vi "Handle Last Ack Core.vi"(4 "error in (no error)":errorcluster, 6 "Last Ack":refnum<class "Last Ack.lvclass">, 7 "ViewableActor in":refnum<class "ViewableActor.lvclass">) -> (0 "error out":errorcluster, 3 "ViewableActor out":refnum<class "ViewableActor.lvclass">)   [LabVIEW 2020, in "ViewableActor.lvlib" / "ViewableActor.lvclass"]
doc: "(<B>Filename</B>: Actor Framework.lvlib:Actor.lvclass:Handle Last Ack Core.vi)\n\nDefines how the caller actor responds to the Last Ack message from a nested actor. The Last Ack message is the final message a nested actor sends to its caller before it shuts down. The message contains information about the final state of the nested actor.\n\nBy default, this method does nothing except return any error the nested actor sent. A descendant class may override this method to define behavior."
uses:
  ViewableActor.lvclass
  <vilib>/ActorFramework/LastAck/Last Ack.lvclass
  Error Display Actor/Error Display Actor.lvclass
  <vilib>/ActorFramework/LastAck/Last Ack.lvclass/Last Ack.ctl
  Error Display Actor/Error Display Actor.lvclass/Error Display Actor.ctl
  ViewableActor.lvclass/ViewableActor.ctl
  Error Display Actor/Read error for msg.vi
  <vilib>/ActorFramework/Actor/Actor.lvclass
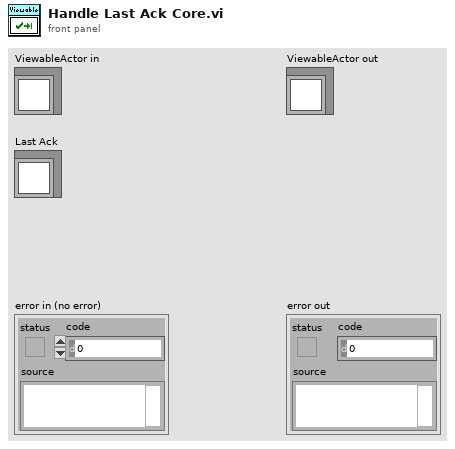
[diagram p1: front panel]
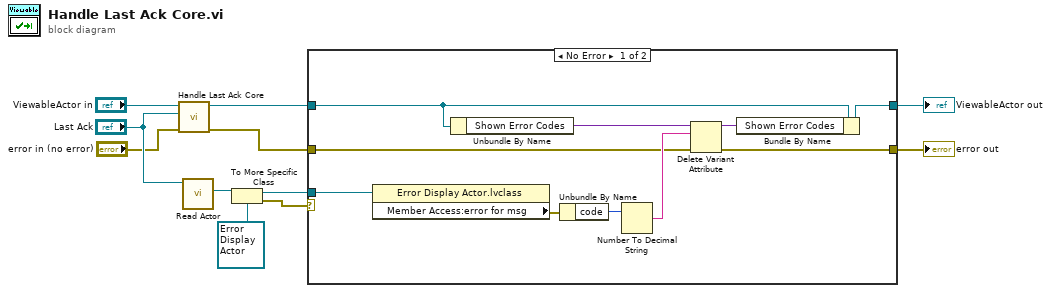
[diagram p0: block diagram]
diagram:
  n1 = call-parent "Handle Last Ack Core.vi"("error in (no error)"="error in (no error)", "Last Ack"="Last Ack", "Actor in"="ViewableActor in") -> ("error out"=w2:errorcluster, "Actor out"=w4:refnum<class "ViewableActor.lvclass">)  [unwired: 3 in]
  n2 = call <vilib>:"Read Actor.vi"("Last Ack"="Last Ack") -> ("Actor"=w8:refnum<class "Actor.lvclass">)  [unwired: 10 in]
  n3 = To More Specific Class(target class=refnum<class "Error Display Actor.lvclass"> refnum ("ViewableActor.lvlib:Error Display Actor.lvclass"), reference=w8) -> (specific class reference=w5:refnum<class "Error Display Actor.lvclass">, error out=w6:errorcluster)  [unwired: 1 in]
  n4 = case shown="No Error" w6 {
    tunnel: w5 -> [w20 _]
    tunnel: w4 -> [w16 w23]
    tunnel: [w15 w23] -> w3
    tunnel: w2 -> [w13 w22]
    tunnel: [w12 w22] -> w1
    frame No Error {
      n5 = property class="Error Display Actor.lvclass"(reference=w20) -> ("Member Access:error for msg"=w19:errorcluster)  [unwired: 1 in, 2 out]
      n6 = Unbundle By Name(w16) -> ("Shown Error Codes"=w21:variant)
      n7 = Unbundle By Name(w19) -> ("code"=w18:i32)
      n8 = Number To Decimal String(number=w18) -> (decimal integer string=w17:string)  [unwired: 1 in]
      n9 = Delete Variant Attribute(4:w13, 6:w17, 7:w21) -> (0:w12:errorcluster, 3:w14:variant)  [unwired: 1 out]
      n10 = Bundle By Name(cluster=w16, "Shown Error Codes"=w14) -> (w15:refnum<class "ViewableActor.lvclass">)
    }
    frame Error {
    }
  }
  "ViewableActor out" <- w3
  "error out" <- w1
